vi "Configure Generator Tracking.vi"(5 "Enable Frequency Tracking (F: Disable)":bool, 6 "Copy Signal (F: Disable)":bool, 7 "Enable Amplitude Tracking (F: Disable)":bool, 8 "error in (no error)":errorcluster, 9 "Enable Tracking (F: Disable)":bool, 10 "Waveform Generator Number (1: Waveform Generator 1)":i32(ring)=1 items=["Waveform Generator 1"=1, "Waveform Generator 2"=2], 11 "VISA resource name":refnum<visa-resource-name>) -> (0 "error out":errorcluster, 3 "VISA resource name out":refnum<visa-resource-name>)   [LabVIEW 2010, in "Agilent 2000 3000 X-Series.lvlib"]
doc: "Configures waveform generator tracking."
uses:
  <instrlib>/Agilent 2000 3000 X-Series/Agilent 2000 3000 X-Series.lvlib
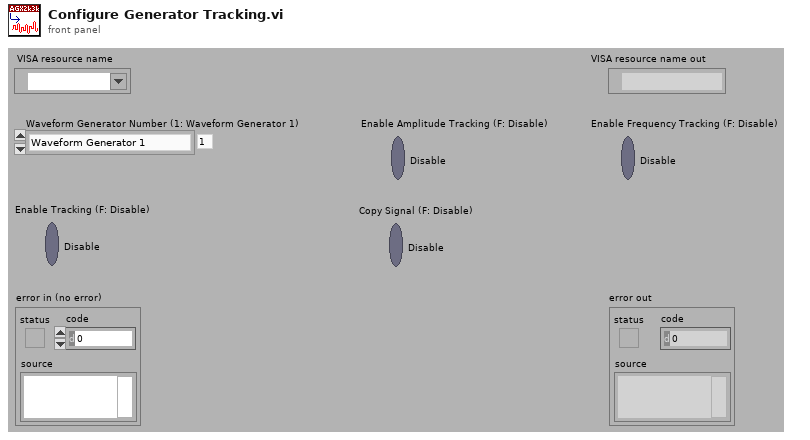
[diagram p1: front panel]
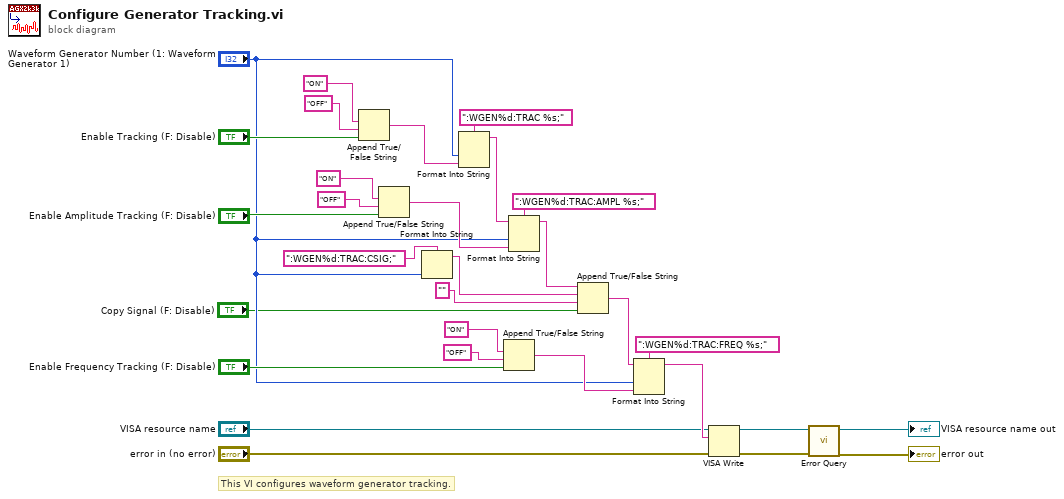
[diagram p0: block diagram]
diagram:
  # "This VI configures waveform generator tracking."
  n1 = Append True/False String(1:"Enable Tracking (F: Disable)", 2:"OFF", 3:"ON") -> (0:w26:string)  [unwired: 1 out]
  n2 = Append True/False String(1:"Enable Amplitude Tracking (F: Disable)", 2:"OFF", 3:"ON") -> (0:w20:string)  [unwired: 1 out]
  n3 = Format Into String(format string=":WGEN%d:TRAC:CSIG;", "Waveform Generator Number (1: Waveform Generator 1)") -> (resulting string=w5:string)  [unwired: 2 in, 1 out]
  n4 = Format Into String(format string=":WGEN%d:TRAC %s;", "Waveform Generator Number (1: Waveform Generator 1)", w26) -> (resulting string=w22:string)  [unwired: 2 in, 1 out]
  n5 = Append True/False String(1:"Enable Frequency Tracking (F: Disable)", 2:"OFF", 3:"ON") -> (0:w15:string)  [unwired: 1 out]
  n6 = Format Into String(format string=":WGEN%d:TRAC:AMPL %s;", initial string=w22, "Waveform Generator Number (1: Waveform Generator 1)", w20) -> (resulting string=w1:string)  [unwired: 1 in, 1 out]
  n7 = Append True/False String(1:"Copy Signal (F: Disable)", 2:"", 3:w5, 4:w1) -> (0:w2:string)
  n8 = Format Into String(format string=":WGEN%d:TRAC:FREQ %s;", initial string=w2, "Waveform Generator Number (1: Waveform Generator 1)", w15) -> (resulting string=w14:string)  [unwired: 1 in, 1 out]
  n9 = VISA Write(VISA resource name="VISA resource name", write buffer=w14, error in (no error)="error in (no error)") -> (VISA resource name out=w11:refnum<visa-resource-name>, error out=w10:errorcluster)  [unwired: 1 out]
  n10 = call <instrlib>:"Error Query.vi"("error in (no error)"=w10, "VISA resource name"=w11) -> ("error out"=→"error out":errorcluster, "VISA resource name out"=→"VISA resource name out":refnum<visa-resource-name>)  [unwired: 8 out]
